vi "Construct.vi"(1 "Cell Size":i16, 2 "Canvas Ref in":refnum<vi>) -> (0 "CollisionGrid.lvclass":refnum<class "CollisionGrid.lvclass">)   [LabVIEW 2022 SP3, in "CollisionGrid.lvclass"]
uses:
  CollisionGrid.lvclass
  CollisionGrid.lvclass/CollisionGrid.ctl
  Math/Vector2/Vector2.lvclass
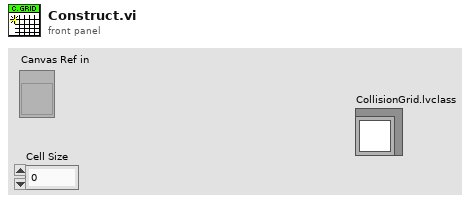
[diagram p1: front panel]
types:
  T1 = typedef "LVBoundsTypeDef.ctl" = cluster{"Width":u32, "Height":u32}
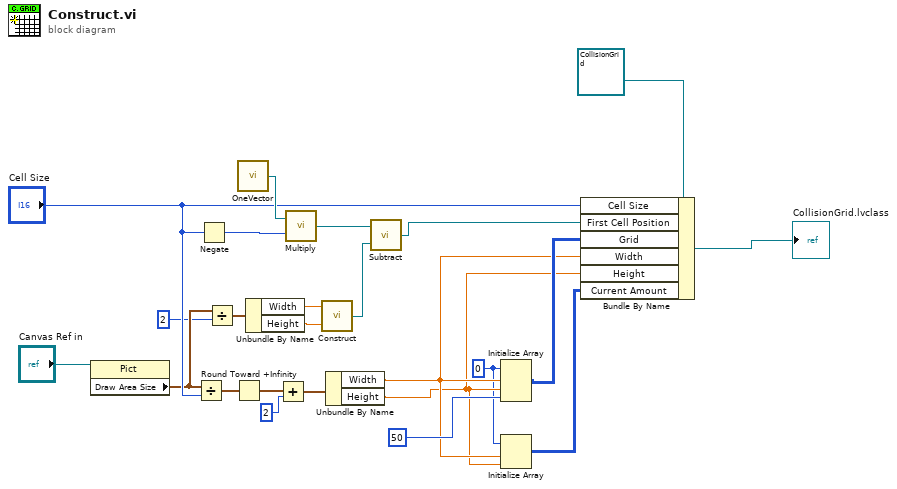
[diagram p0: block diagram]
diagram:
  w2 = i16 0 ("element")
  n1 = property class="Pict"(reference="Canvas Ref in") -> ("Draw Area Size"=w6:T1)  [unwired: 1 in, 2 out]
  n2 = Divide(x=w6, y="Cell Size") -> (x/y=w13:cluster{"Width":dbl, "Height":dbl})
  n3 = Negate(x="Cell Size") -> (-x=w15:i16)
  n4 = Divide(x=w6, y=2) -> (x/y=w7:cluster{"Width":dbl, "Height":dbl})
  n5 = Round Toward +Infinity(x=w13) -> (ceil(x): smallest int >= x=w22:cluster{"Width":dbl, "Height":dbl})
  n6 = call "OneVector.vi"() -> ("One Vector"=w19:refnum<class "Vector2.lvclass">)
  n7 = Unbundle By Name(w7) -> ("Width"=w12:dbl, "Height"=w11:dbl)
  n8 = Add(x=w22, y=2) -> (x+y=w18:cluster{"Width":dbl, "Height":dbl})
  n9 = call "Multiply.vi"("Scalar"=w15, "Vector in"=w19) -> ("Vector out"=w10:refnum<class "Vector2.lvclass">)
  n10 = call "Construct.vi"("y"=w11, "x"=w12) -> ("Vec2 out"=w9:refnum<class "Vector2.lvclass">)
  n11 = Unbundle By Name(w18) -> ("Width"=w4:dbl, "Height"=w3:dbl)
  n12 = call "Subtract.vi"("Vec2 b in"=w9, "Vec2 a in"=w10) -> ("Vec2 out"=w8:refnum<class "Vector2.lvclass">)
  n13 = Initialize Array(w2, w4, w3, i8 50 ("dimension size")) -> (w16:i16[][][])
  n14 = Initialize Array(w2, w4, w3) -> (w1:i16[][])
  n15 = Bundle By Name(cluster=refnum<class "CollisionGrid.lvclass"> refnum ("CollisionGrid.lvclass"), "Cell Size"="Cell Size", "First Cell Position"=w8, "Grid"=w16, "Width"=w4, "Height"=w3, "Current Amount"=w1) -> (→"CollisionGrid.lvclass":refnum<class "CollisionGrid.lvclass">)
